vi "OFFINISH_parse_PLC.vi"(11 "String":string="OFFINISHOK200084480_A|1|PCS||00001|$R") -> (2 "OF":string, 3 "étage":string)   [LabVIEW 2020]
uses:
  <vilib>/regexp/Match Regular Expression.xnode
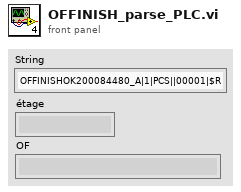
[diagram p1: front panel]
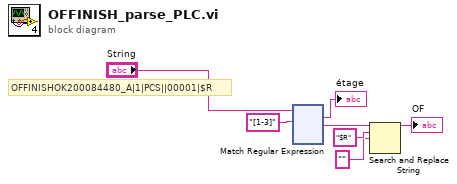
[diagram p0: block diagram]
diagram:
  # "OFFINISHOK200084480_A|1|PCS||00001|$R"
  n1 = xnode "Match Regular Expression"("input string"="String", "regular expression"="[1-3]") -> ("whole match"=→"étage":string, "after match"=w4:string)  [unwired: 4 in, 3 out]
  n2 = Search and Replace String(input string=w4, search string="$R" ("substring (\"\")"), replace string="" ("replace string (\"\")")) -> (result string=→"OF":string)  [unwired: 5 in, 3 out]
